vi "Initialize.vi"(8 "error in (no error)":errorcluster, 9 "Plugin Folder":path, 11 "File Parser Interface in":refnum<class "File Parser Interface.lvclass">) -> (0 "error out":errorcluster, 3 "File Parser Interface out":refnum<class "File Parser Interface.lvclass">)   [LabVIEW 2018, in "File Parser Interface.lvlib" / "File Parser Interface.lvclass"]
uses:
  File Parser Interface.lvclass
  File Parser Interface.lvclass/File Parser Interface.ctl
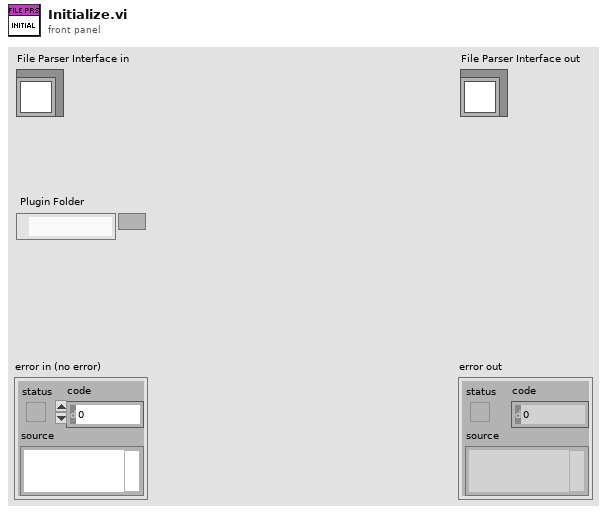
[diagram p1: front panel]
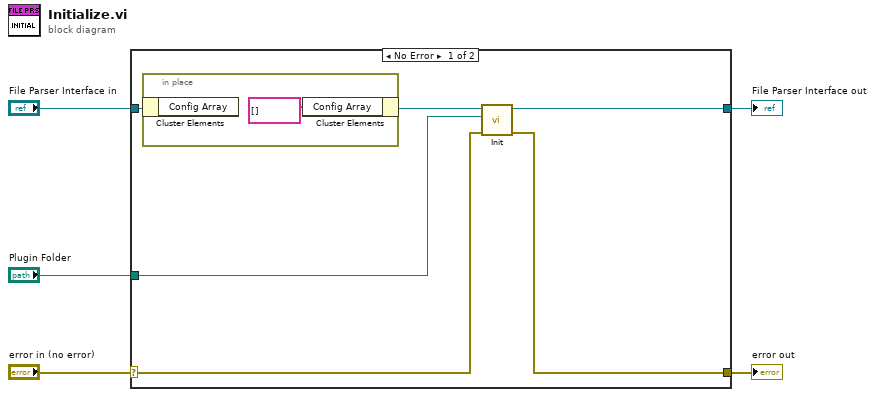
[diagram p0: block diagram]
diagram:
  n1 = case shown="No Error" "error in (no error)" {
    selector: "error in (no error)" -> [w7 w14]
    tunnel: [w6 w14] -> w4
    tunnel: [w9 w13] -> w2
    tunnel: "File Parser Interface in" -> [w11 w13]
    tunnel: "Plugin Folder" -> [w8 _]
    frame No Error {
      n2 = in-place {
        n3 = in-place-cluster #1(w11) -> ()  [unwired: 1 out]
        n4 = in-place-cluster #1("Config Array"=string[] []) -> (w10:refnum<class "File Parser Interface.lvclass">)
      }
      n5 = call-dynamic "Init.vi"("Error In"=w7, "Folder Path"=w8, "Plugin Framework In"=w10) -> ("Error Out"=w6:errorcluster, "File Parser Interface out"=w9:refnum<class "File Parser Interface.lvclass">)  [unwired: 7 in]
    }
    frame Error {
    }
  }
  "error out" <- w4
  "File Parser Interface out" <- w2
